vi "Un(Re)doTblChng.vi"(4 "Defer Updates?":bool=TRUE, 5 "Undo/Redo":enum16{"Undo", "Redo"}(ring), 6 "ModeCol Index":i32=2, 7 "Layout Ref":refnum<vi>, 8 "error in (no error)":errorcluster, 9 "Table CtlRef In":refnum<vi>, 10 "Col Array in":refnum<class "Column.lvclass">[](array[class]), 11 "Table History ref":refnum<vi>) -> (0 "error out":errorcluster)   [LabVIEW 2013]
doc: "Depending on Undo/Redo enum:\n undo: Swap current Table with older History + increment internal pointer;\n redo: decrement internal pointer + swap current Table with newer History.\n\nThis VI is read-only w.r.t Column Array."
uses:
  TypeDefs/TableHistory.ctl
  TypeDefs/TableArray.ctl
  ColumnVIs/Column/Column.lvclass
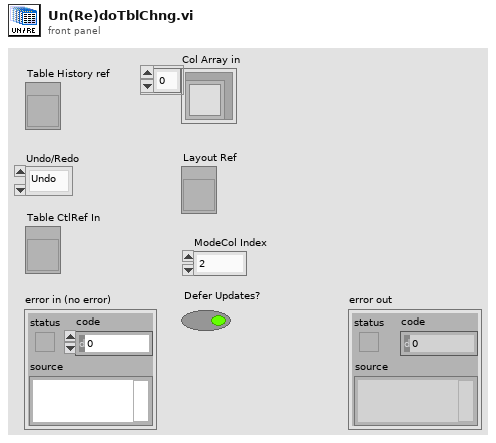
[diagram p1: front panel]
types:
  T1 = typedef "TableHistory.ctl" = cluster{"OldTable Array":T2, "Undo pointer":i32}
  T2 = typedef "TableArray.ctl" = cluster{"OldTable":string[][]}[]
  T3 = typedef "LVRowAndColumnTypeDef.ctl" = cluster{"Row":i32, "Column":i32}
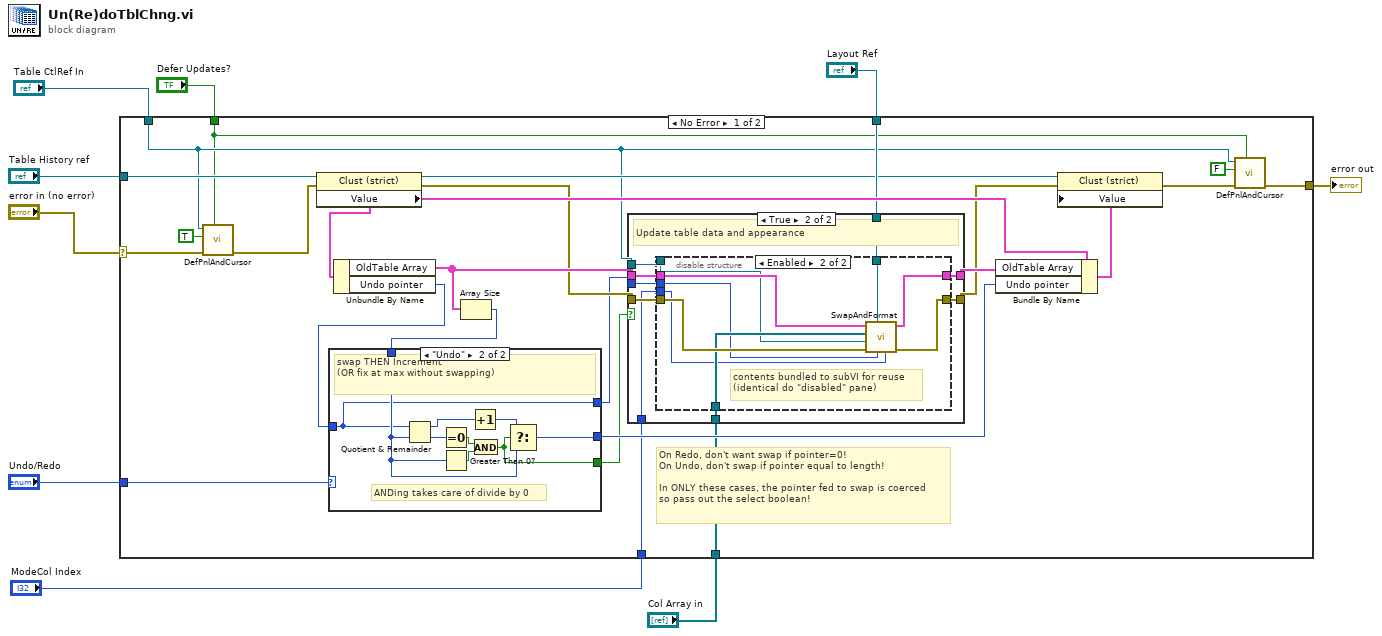
[diagram p0: block diagram]
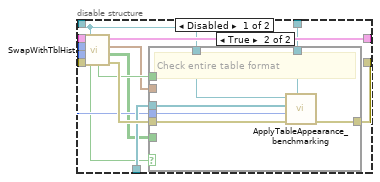
[diagram p3: hidden frame]
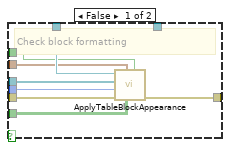
[diagram p4: hidden frame]
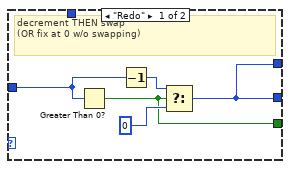
[diagram p5: hidden frame]
diagram:
  n1 = case shown="No Error" "error in (no error)" {
    selector: "error in (no error)" -> [w15 w97]
    tunnel: "Undo/Redo" -> [w34 _]
    tunnel: "Table History ref" -> [w33 _]
    tunnel: [w12 w97] -> w7
    tunnel: "Table CtlRef In" -> [w11 _]
    tunnel: "Col Array in" -> [w19 _]
    tunnel: "Layout Ref" -> [w20 _]
    tunnel: "ModeCol Index" -> [w21 _]
    tunnel: "Defer Updates?" -> [w10 _]
    frame No Error {
      # "On Redo, don't want swap if pointer=0!\nOn Undo, don't swap if pointer equal to length!\n\nIn ONLY these cases, the pointer fed to swap is coerced\nso pass out the select boolean!"
      n2 = call "DefPnlAndCursor.vi"("AllowDefPan? (T)"=w10, "error in (no error)"=w15, "DeferPanUpdts?"=TRUE ("DeferPanUPdts?"), "Tbl Ctrl Refnum"=w11) -> ("error out"=w16:errorcluster)  [unwired: 7 in]
      n3 = property class="Clust (strict)"(reference=w33, error in=w16) -> (reference out=w18:refnum<vi>, error out=w26:errorcluster, "Value"=w31:T1)
      n4 = Unbundle By Name(w31) -> ("OldTable Array"=w28:T2, "Undo pointer"=w23:i32)
      n5 = Array Size(array=w28) -> (size(s)=w32:i32)
      n6 = case shown="\"Undo\"" w34 {
        tunnel: w23 -> [w86 w89]
        tunnel: [w84 w93] -> w29
        tunnel: [w84 w89] -> w24
        tunnel: w32 -> [_ w92]
        tunnel: [w83 w88] -> w22
        frame "Redo" {
          # "decrement THEN swap\n(OR fix at 0 w/o swapping)"
          n7 = Greater Than 0?(x=w86) -> (x > 0?=w83:bool)
          n8 = Decrement(x=w86) -> (x-1=w85:i32)
          n9 = Select(t=w85, s=w83, f=0) -> (s? t:f=w84:i32)
        }
        frame "Undo" {
          # "ANDing takes care of divide by 0"
          # "swap THEN Increment\n(OR fix at max without swapping)"
          n10 = Quotient & Remainder(x=w89, y=w92) -> (x-y*floor(x/y)=w95:i32, floor(x/y)=w96:i32)
          n11 = Equal To 0?(x=w96) -> (x = 0?=w91:bool)
          n12 = Greater Than 0?(x=w92) -> (x > 0?=w90:bool)
          n13 = Increment(x=w95) -> (x+1=w94:i32)
          n14 = And(x=w91, y=w90) -> (x .and. y?=w88:bool)
          n15 = Select(t=w94, s=w88, f=w92) -> (s? t:f=w93:i32)
        }
      }
      n16 = case shown="True" w22 {
        tunnel: w28 -> [w36 w45]
        tunnel: [w36 w44] -> w27
        tunnel: w26 -> [w35 w43]
        tunnel: [w35 w41] -> w25
        tunnel: w24 -> [_ w42]
        tunnel: w11 -> [_ w40]
        tunnel: w21 -> [_ w37]
        tunnel: w20 -> [_ w39]
        tunnel: w19 -> [_ w38]
        frame False {
          # "at oldest/newest change: do nothing!"
        }
        frame True {
          # "Update table data and appearance"
          n17 = disable-structure shown="Enabled" {
            disable-tunnel: w45 -> [w59 w79]
            disable-tunnel: [w58 w78] -> w44
            disable-tunnel: w43 -> [w57 w81]
            disable-tunnel: w42 -> [w56 w75]
            disable-tunnel: [w54 w82] -> w41
            disable-tunnel: w40 -> [w53 w76]
            disable-tunnel: w39 -> [w52 w77]
            disable-tunnel: w38 -> [w51 w80]
            disable-tunnel: w37 -> [w50 w74]
            frame Disabled {
              n18 = call "SwapWithTblHist.vi"("Table CtlRef In"=w53, "error in (no error)"=w57, "Mode Index"=w50, "Undo pointer"=w56, "OldTable Array in"=w59) -> ("error out"=w55:errorcluster, "changed? subarray"=w47:bool[][], "Change start"=w46:T3, "OldTable Array out"=w58:T2, "Mode change?"=w48:bool, "Size mismatch?"=w49:bool)  [unwired: 1 in]
              n19 = case shown="True" w49 {
                tunnel: w55 -> [w67 w73]
                tunnel: [w66 w72] -> w54
                tunnel: w53 -> [w65 w71]
                tunnel: w52 -> [_ w70]
                tunnel: w51 -> [w64 w69]
                tunnel: w50 -> [w63 w68]
                tunnel: w48 -> [w62 _]
                tunnel: w47 -> [w61 _]
                tunnel: w46 -> [w60 _]
                frame False {
                  # "Check block formatting"
                  n20 = call "ApplyTableBlockAppearance.vi"("Check Mode?"=w62, "changed? subarray"=w61, "Change start"=w60, "error in (no error)"=w67, "Mode Index"=w63, "Col Array in"=w64, "Table Ref in"=w65) -> ("error out"=w66:errorcluster)  [unwired: 4 in]
                }
                frame True {
                  # "Check entire table format"
                  n21 = call "ApplyTableAppearance_benchmarking.vi"("Layout Ring Ref"=w70, "error in (no error)"=w73, "Mode Index"=w68, "Col Array in"=w69, "Table Ref in"=w71) -> ("error out"=w72:errorcluster)  [unwired: 5 in, 1 out]
                }
              }
            }
            frame Enabled {
              # "contents bundled to subVI for reuse\n(identical do \"disabled\" pane)"
              n22 = call "SwapAndFormat.vi"("Mode Index"=w74, "Undo pointer"=w75, "Layout Ref"=w77, "error in (no error)"=w81, "Table CtlRef In"=w76, "Col Array in"=w80, "OldTable Array in"=w79) -> ("error out"=w82:errorcluster, "OldTable Array out"=w78:T2)  [unwired: 3 in]
            }
          }
        }
      }
      n23 = Bundle By Name(cluster=w31, "OldTable Array"=w27, "Undo pointer"=w29) -> (w30:T1)
      n24 = property class="Clust (strict)"(reference=w18, error in=w25, "Value"=w30) -> (error out=w13:errorcluster)  [unwired: 1 out]
      n25 = call "DefPnlAndCursor.vi"("AllowDefPan? (T)"=w10, "error in (no error)"=w13, "DeferPanUpdts?"=FALSE ("DeferPanUPdts?"), "Tbl Ctrl Refnum"=w11) -> ("error out"=w12:errorcluster)  [unwired: 7 in]
    }
    frame Error {
    }
  }
  "error out" <- w7
